vi "Read Core.vi"(8 "error in (no error)":errorcluster, 9 "Timeout (1s)":dbl[unit]=1.0, 11 "PVConnection in":refnum<class "PVConnection.lvclass">) -> (0 "error out":errorcluster, 1 "timed out":bool, 2 "PV":refnum<class "PV.lvclass">, 3 "PVConnection out":refnum<class "PVConnection.lvclass">)   [LabVIEW 2015, in "CS++ProcessVariables.lvlib" / "PVConnection.lvclass"]
doc: "Read a process variable."
uses:
  PVConnection.lvclass
  ProcessVariable/PV.lvclass
  PVConnection.lvclass/PVConnection.ctl
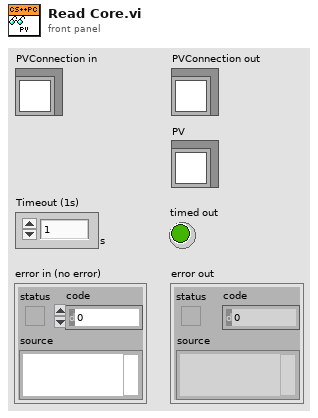
[diagram p1: front panel]
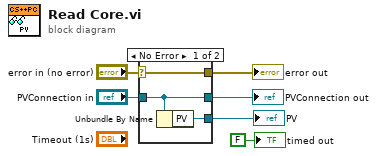
[diagram p0: block diagram]
diagram:
  n1 = case shown="No Error" "error in (no error)" {
    selector: "error in (no error)" -> [w9 w11]
    tunnel: [w9 w11] -> w5
    tunnel: [w8 w10] -> w3
    tunnel: "PVConnection in" -> [w8 w10]
    tunnel: [w7 _] -> w2
    frame No Error {
      n2 = Unbundle By Name(w8) -> ("PV"=w7:refnum<class "PV.lvclass">)
    }
    frame Error {
    }
  }
  "error out" <- w5
  "PVConnection out" <- w3
  "PV" <- w2
  "timed out" <- FALSE ("timed out")
